vi "Variant_to_Array.vi"(8 "Error in":errorcluster, 11 "Value (in)":variant) -> (0 "Error out":errorcluster, 2 "Value (string)":string, 3 "Value (out)":string)   [LabVIEW 2012]
uses:
  Variant_to_I8.vi
  Variant_to_I16.vi
  Variant_to_I32.vi
  Variant_to_I64.vi
  Variant_to_U8.vi
  Variant_to_U16.vi
  Variant_to_U32.vi
  Variant_to_U64.vi
  Variant_to_SGL.vi
  Variant_to_DBL.vi
  Variant_to_EXT.vi
  Variant_to_CSG.vi
  Variant_to_CDB.vi
  Variant_to_CXT.vi
  Variant_to_Enum_U8.vi
  Variant_to_Enum_U16.vi
  Variant_to_Enum_U32.vi
  Variant_to_Enum_U64.vi
  Variant_to_Boolean.vi
  Variant_to_String.vi
  Variant_to_Path.vi
  Variant_to_Cluster.vi
  Variant_to_Waveform_info.vi
  Variant_to_Timestamp.vi
  Variant_to_Refnum.vi
  Variant_to_Fixed_point.vi
  <vilib>/Utility/VariantDataType/VariantType.lvlib
  Variant_to_Waveform.vi
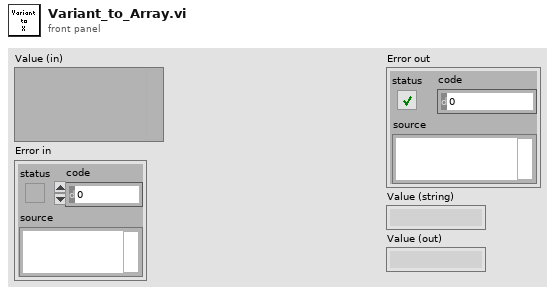
[diagram p1: front panel]
types:
  T1 = typedef "VariantType.lvlib/Type.ctl" = enum8{"Invalid Type", "Void", "I8", "I16", "I32", "I64", "U8", "U16", "U32", "U64", "Single Float", "Double Float", "Extended Float", "Single Complex", "Double Complex", "Extended Complex", "Enum U8", "Enum U16", "Enum U32", "Enum U64", "Single Float With Unit", "Double Float With Unit", "Extended Float With Unit", "Single Complex with Unit", "Double Complex with Unit", "Extended Complex with Unit", "Boolean", "String", "Path", "Picture", "Tag", "Array", "Cluster", "Variant", "LV Variant", "Waveform", "Timestamp", "Digital Waveform", "Digital Data", "ExpressData", "Refnum", "External Data", "VI", "Poly VI", "LabVIEW Class Instance", "Fixed Point"}
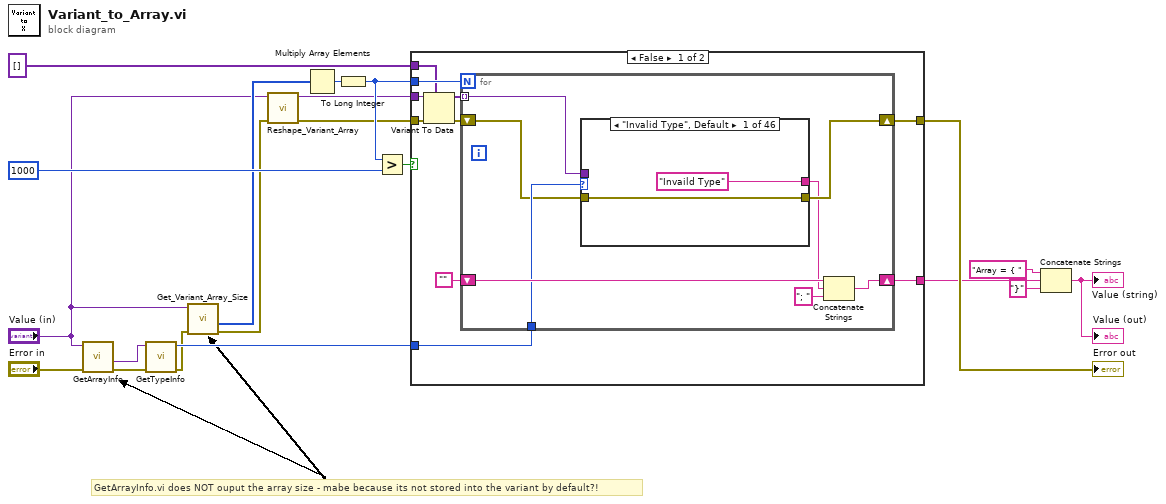
[diagram p0: block diagram]
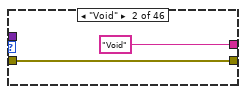
[diagram p2: hidden frame]
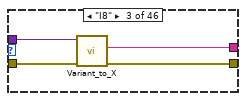
[diagram p3: hidden frame]
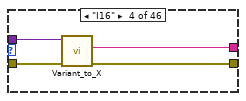
[diagram p4: hidden frame]
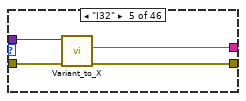
[diagram p5: hidden frame]
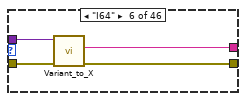
[diagram p6: hidden frame]
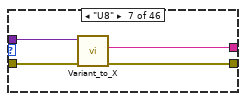
[diagram p7: hidden frame]
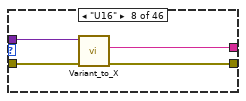
[diagram p8: hidden frame]
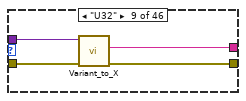
[diagram p9: hidden frame]
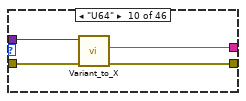
[diagram p10: hidden frame]
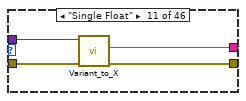
[diagram p11: hidden frame]
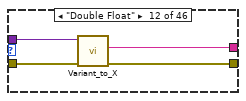
[diagram p12: hidden frame]
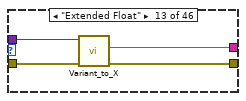
[diagram p13: hidden frame]
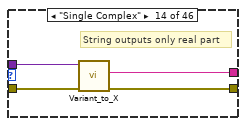
[diagram p14: hidden frame]
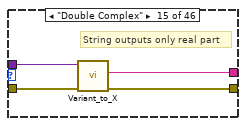
[diagram p15: hidden frame]
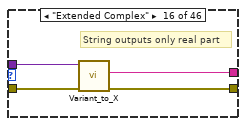
[diagram p16: hidden frame]
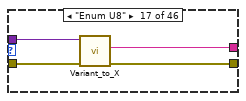
[diagram p17: hidden frame]
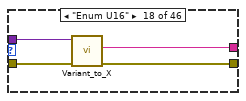
[diagram p18: hidden frame]
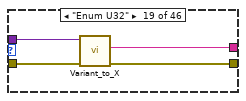
[diagram p19: hidden frame]
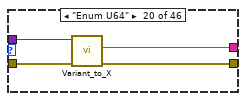
[diagram p20: hidden frame]
diagram:
  # "GetArrayInfo.vi does NOT ouput the array size - mabe because its not stored into the variant by default?!"
  n1 = call <vilib>:"GetArrayInfo.vi"("error in (no error)"="Error in", "Variant"="Value (in)") -> ("error out"=w20:errorcluster, "ArrayElement"=w17:variant)  [unwired: 6 in, 2 out]
  n2 = call <vilib>:"GetTypeInfo.vi"("error in (no error)"=w20, "Variant"=w17) -> ("error out"=w6:errorcluster, "Type Enum"=w19:T1)  [unwired: 5 in, 3 out]
  n3 = call "Get_Variant_Array_Size.vi"("error in (no error)"=w6, "Array in"="Value (in)") -> ("error out"=w4:errorcluster, "Size(s)"=w7:u32[])  [unwired: 6 in, 2 out]
  n4 = call "Reshape_Variant_Array.vi"("error in (no error)"=w4, "MultiD Array"="Value (in)") -> ("error out"=w2:errorcluster, "1D VArray"=w3:variant)  [unwired: 8 in]
  n5 = Multiply Array Elements(1:w7) -> (0:w11:u32)
  n6 = To Long Integer(number=w11) -> (32bit integer=w9:i32)
  n7 = Greater?(x=w9, y=1000) -> (0:w8:bool)
  n8 = case shown="False" w8 {
    tunnel: w19 -> [w30 _]
    tunnel: [w28 w193] -> w16
    tunnel: w3 -> [w25 _]
    tunnel: w2 -> [w24 w193]
    tunnel: [w27 w194] -> w13
    tunnel: w9 -> [w26 w198]
    tunnel: variant[] [] -> [w21 _]
    frame False {
      n9 = Variant To Data(error in=w24, type=w21, Variant=w25) -> (data=w23:variant[], error out=w22:errorcluster)
      n10 = for {
        N: w26 -> [_]
        tunnel: w30 -> [w35]
        tunnel: w23 -> [w32] mode=indexing
        shift-right: [w34] -> w28
        shift-left: w22 -> [w31]
        shift-right: [w37] -> w27
        shift-left: "" -> [w38]
        n11 = case shown="\"Invalid Type\", Default" w35 {
          tunnel: ["Invaild Type" "Void" w44 w47 w51 w55 w59 w63 w67 w72 w76 w79 w83 w87 w91 w95 w99 w104 w107 w111 "{Single Float With Unit}" "{Double Float With Unit}" "{Extended Float With Unit}" "{Single Complex with Unit}" "{Double Complex with Unit}" "{Extended Complex with Unit}" w127 w131 w135 "{Picture}" "{Tag}" w143 w147 "{Variant}" "{LV Variant}" w155 w167 "{Digital Wavefrom}" "{Digital Data}" "{ExpressData}" w177 "{External Data}" "{VI}" "{Poly VI}" "{LabVIEW Class Instance}" w189] -> w33
          tunnel: w32 -> [_ _ w46 w50 w54 w58 w62 w66 w70 w74 w78 w80 w86 w90 w94 w96 w102 w106 w110 w114 _ _ _ _ _ _ w130 w134 w138 _ _ w144 w150 _ _ w158 w170 _ _ _ w180 _ _ _ _ w192]
          tunnel: w31 -> [w39 w41 w45 w49 w53 w57 w61 w65 w69 w73 w77 w82 w85 w89 w93 w98 w101 w105 w109 w113 w116 w118 w120 w122 w124 w126 w129 w133 w137 w140 w142 w146 w149 w152 w154 w157 w169 w171 w174 w176 w179 w182 w184 w186 w188 w191]
          tunnel: [w39 w41 w43 w48 w52 w56 w60 w64 w68 w71 w75 w81 w84 w88 w92 w97 w100 w103 w108 w112 w116 w118 w120 w122 w124 w126 w128 w132 w136 w140 w142 w145 w148 w152 w154 w156 w168 w171 w174 w176 w178 w182 w184 w186 w188 w190] -> w34
          frame "Invalid Type", Default {
          }
          frame "Void" {
          }
          frame "I8" {
            n12 = call-poly "Variant_to_X.vi"("Error in"=w45, "Value (in)"=w46) -> ("Error out"=w43:errorcluster, "Value (string)"=w44:string)  [unwired: 7 in, 1 out]
          }
          frame "I16" {
            n13 = call-poly "Variant_to_X.vi"("Error in"=w49, "Value (in)"=w50) -> ("Error out"=w48:errorcluster, "Value (string)"=w47:string)  [unwired: 7 in, 1 out]
          }
          frame "I32" {
            n14 = call-poly "Variant_to_X.vi"("Error in"=w53, "Value (in)"=w54) -> ("Error out"=w52:errorcluster, "Value (string)"=w51:string)  [unwired: 7 in, 1 out]
          }
          frame "I64" {
            n15 = call-poly "Variant_to_X.vi"("Error in"=w57, "Value (in)"=w58) -> ("Error out"=w56:errorcluster, "Value (string)"=w55:string)  [unwired: 7 in, 1 out]
          }
          frame "U8" {
            n16 = call-poly "Variant_to_X.vi"("Error in"=w61, "Value (in)"=w62) -> ("Error out"=w60:errorcluster, "Value (string)"=w59:string)  [unwired: 7 in, 1 out]
          }
          frame "U16" {
            n17 = call-poly "Variant_to_X.vi"("Error in"=w65, "Value (in)"=w66) -> ("Error out"=w64:errorcluster, "Value (string)"=w63:string)  [unwired: 7 in, 1 out]
          }
          frame "U32" {
            n18 = call-poly "Variant_to_X.vi"("Error in"=w69, "Value (in)"=w70) -> ("Error out"=w68:errorcluster, "Value (string)"=w67:string)  [unwired: 7 in, 1 out]
          }
          frame "U64" {
            n19 = call-poly "Variant_to_X.vi"("Error in"=w73, "Value (in)"=w74) -> ("Error out"=w71:errorcluster, "Value (string)"=w72:string)  [unwired: 7 in, 1 out]
          }
          frame "Single Float" {
            n20 = call-poly "Variant_to_X.vi"("Error in"=w77, "Value (in)"=w78) -> ("Error out"=w75:errorcluster, "Value (string)"=w76:string)  [unwired: 7 in, 1 out]
          }
          frame "Double Float" {
            n21 = call-poly "Variant_to_X.vi"("Error in"=w82, "Value (in)"=w80) -> ("Error out"=w81:errorcluster, "Value (string)"=w79:string)  [unwired: 7 in, 1 out]
          }
          frame "Extended Float" {
            n22 = call-poly "Variant_to_X.vi"("Error in"=w85, "Value (in)"=w86) -> ("Error out"=w84:errorcluster, "Value (string)"=w83:string)  [unwired: 7 in, 1 out]
          }
          frame "Single Complex" {
            # "String outputs only real part"
            n23 = call-poly "Variant_to_X.vi"("Error in"=w89, "Value (in)"=w90) -> ("Error out"=w88:errorcluster, "Value (string)"=w87:string)  [unwired: 7 in, 1 out]
          }
          frame "Double Complex" {
            # "String outputs only real part"
            n24 = call-poly "Variant_to_X.vi"("Error in"=w93, "Value (in)"=w94) -> ("Error out"=w92:errorcluster, "Value (string)"=w91:string)  [unwired: 7 in, 1 out]
          }
          frame "Extended Complex" {
            # "String outputs only real part"
            n25 = call-poly "Variant_to_X.vi"("Error in"=w98, "Value (in)"=w96) -> ("Error out"=w97:errorcluster, "Value (string)"=w95:string)  [unwired: 7 in, 1 out]
          }
          frame "Enum U8" {
            n26 = call-poly "Variant_to_X.vi"("Error in"=w101, "Value (in)"=w102) -> ("Error out"=w100:errorcluster, "Value (string)"=w99:string)  [unwired: 7 in, 1 out]
          }
          frame "Enum U16" {
            n27 = call-poly "Variant_to_X.vi"("Error in"=w105, "Value (in)"=w106) -> ("Error out"=w103:errorcluster, "Value (string)"=w104:string)  [unwired: 7 in, 1 out]
          }
          frame "Enum U32" {
            n28 = call-poly "Variant_to_X.vi"("Error in"=w109, "Value (in)"=w110) -> ("Error out"=w108:errorcluster, "Value (string)"=w107:string)  [unwired: 7 in, 1 out]
          }
          frame "Enum U64" {
            n29 = call-poly "Variant_to_X.vi"("Error in"=w113, "Value (in)"=w114) -> ("Error out"=w112:errorcluster, "Value (string)"=w111:string)  [unwired: 7 in, 1 out]
          }
          frame "Single Float With Unit" {
          }
          frame "Double Float With Unit" {
          }
          frame "Extended Float With Unit" {
          }
          frame "Single Complex with Unit" {
          }
          frame "Double Complex with Unit" {
          }
          frame "Extended Complex with Unit" {
          }
          frame "Boolean" {
            n30 = call-poly "Variant_to_X.vi"("Error in"=w129, "Value (in)"=w130) -> ("Error out"=w128:errorcluster, "Value (string)"=w127:string)  [unwired: 7 in, 1 out]
          }
          frame "String" {
            n31 = call-poly "Variant_to_X.vi"("Error in"=w133, "Value (in)"=w134) -> ("Error out"=w132:errorcluster, "Value (string)"=w131:string)  [unwired: 7 in, 1 out]
          }
          frame "Path" {
            n32 = call-poly "Variant_to_X.vi"("Error in"=w137, "Value (in)"=w138) -> ("Error out"=w136:errorcluster, "Value (string)"=w135:string)  [unwired: 7 in, 1 out]
          }
          frame "Picture" {
          }
          frame "Tag" {
          }
          frame "Array" {
            n33 = call-poly "Variant_to_X.vi"("Error in"=w146, "Value (in)"=w144) -> ("Error out"=w145:errorcluster, "Value (string)"=w143:string)  [unwired: 7 in, 1 out]
          }
          frame "Cluster" {
            n34 = call-poly "Variant_to_X.vi"("Error in"=w149, "Value (in)"=w150) -> ("Error out"=w148:errorcluster, "Value (string)"=w147:string)  [unwired: 7 in, 1 out]
          }
          frame "Variant" {
          }
          frame "LV Variant" {
          }
          frame "Waveform" {
            n35 = disable-structure shown="Enabled" {
              disable-tunnel: w158 -> [w162 w166]
              disable-tunnel: w157 -> [w161 w165]
              disable-tunnel: [w160 w164] -> w156
              disable-tunnel: [w159 w163] -> w155
              frame Disabled {
                n36 = call-poly "Variant_to_X.vi"("Error in"=w161, "Value (in)"=w162) -> ("Error out"=w160:errorcluster, "Value (string)"=w159:string)  [unwired: 7 in, 1 out]
              }
              frame Enabled {
                n37 = call-poly "Variant_to_X.vi"("Error in"=w165, "Value (in)"=w166) -> ("Error out"=w164:errorcluster, "Value (string)"=w163:string)  [unwired: 7 in, 1 out]
              }
            }
          }
          frame "Timestamp" {
            n38 = call-poly "Variant_to_X.vi"("Error in"=w169, "Value (in)"=w170) -> ("Error out"=w168:errorcluster, "Value (string)"=w167:string)  [unwired: 7 in, 1 out]
          }
          frame "Digital Waveform" {
          }
          frame "Digital Data" {
          }
          frame "ExpressData" {
          }
          frame "Refnum" {
            n39 = call-poly "Variant_to_X.vi"("Error in"=w179, "Value (in)"=w180) -> ("Error out"=w178:errorcluster, "Value (string)"=w177:string)  [unwired: 5 in, 3 out]
          }
          frame "External Data" {
          }
          frame "VI" {
          }
          frame "Poly VI" {
          }
          frame "LabVIEW Class Instance" {
          }
          frame "Fixed Point" {
            n40 = call-poly "Variant_to_X.vi"("Error in"=w191, "Value (in)"=w192) -> ("Error out"=w190:errorcluster, "Value (string)"=w189:string)  [unwired: 7 in, 1 out]
          }
        }
        n41 = Concatenate Strings(w38, w33, "; " ("string")) -> (w37:string)
      }
    }
    frame True {
      # "If there are to many elements in the array, just output the number of elements"
      n42 = Number To Decimal String(number=w198) -> (decimal integer string=w195:string)  [unwired: 1 in]
      n43 = Concatenate Strings("[" ("string"), w195, "] " ("string")) -> (w194:string)
    }
  }
  "Error out" <- w16
  n44 = Concatenate Strings("Array = { " ("string"), w13, "}" ("string")) -> (→"Value (out)" →"Value (string)":string)
